vi "Read chess.vi"(1 "Array":i32[][](array[numeric])) -> (0 "Array 2":i32[][](array[numeric]))   [LabVIEW 2009]
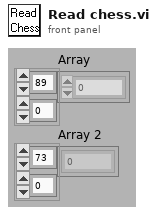
[diagram p1: front panel]
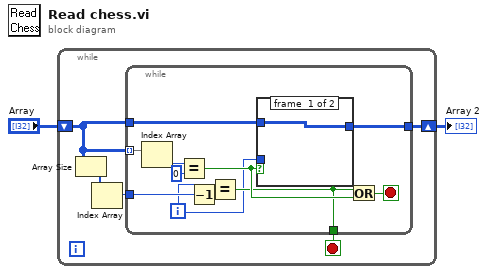
[diagram p0: block diagram]
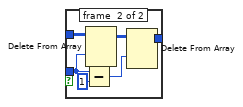
[diagram p2: hidden frame]
diagram:
  n1 = while {
    shift-right: [w7] -> w2
    shift-left: "Array" -> [w3]
    stop <- w4 stop-if-true
    n2 = Array Size(array=w3) -> (size(s)=w6:i32[])
    n3 = Index Array(array=w6) -> (element=w5:i32)  [unwired: 1 in]
    n4 = while {
      tunnel: w3 -> [w16] mode=indexing
      tunnel: w3 -> [w15]
      tunnel: [w14] -> w7
      tunnel: w5 -> [w13]
      tunnel: [w10] -> w4
      i -> [w8]
      stop <- w11 stop-if-true
      n5 = Index Array(array=w16) -> (element=w18:i32)  [unwired: 1 in]
      n6 = Equal?(x=w18, y=0) -> (x = y?=w12:bool)
      n7 = Decrement(x=w13) -> (x-1=w9:i32)
      n8 = Equal?(x=w8, y=w9) -> (x = y?=w10:bool)
      n9 = case shown="True" w12 {
        tunnel: w8 -> [_ w24]
        tunnel: w15 -> [w19 w25]
        tunnel: [w19 w20] -> w14
        frame #0 {
        }
        frame #1 {
          n10 = Subtract(x=w24, y=1) -> (x-y=w21:i32)
          n11 = Delete From Array(array=w25, index (row)=w24) -> (array with subset deleted=w22:i32[][])  [unwired: 2 in, 1 out]
          n12 = Delete From Array(array=w22, index (row)=w21) -> (array with subset deleted=w20:i32[][])  [unwired: 2 in, 1 out]
        }
      }
      n13 = Or(x=w10, y=w12) -> (x .or. y?=w11:bool)
    }
  }
  "Array 2" <- w2
